vi "start.vi"(8 "error in (no error)":errorcluster, 11 "control references in":T1) -> (0 "error out":errorcluster, 3 "control references out":T1)   [LabVIEW 2010]
uses:
  type_definitions/clusters/controls_refs.ctl
  type_definitions/enumerations/main_control_types.ctl
  common/classes/GenericToplevelComponent/GenericToplevelComponent/GenericToplevelComponent.lvclass
  components/ImagingMode/GenericImagingMode/GenericImagingMode/GenericImagingMode.lvclass
  components/ExperimentController/GenericExperimentController/GenericExperimentController/GenericExperimentController.lvclass
  global_variables.vi
  common/classes/GenericComponent/GenericComponent/class_data.vi
  common/classes/GenericComponent/GenericComponent/GenericComponent.lvclass
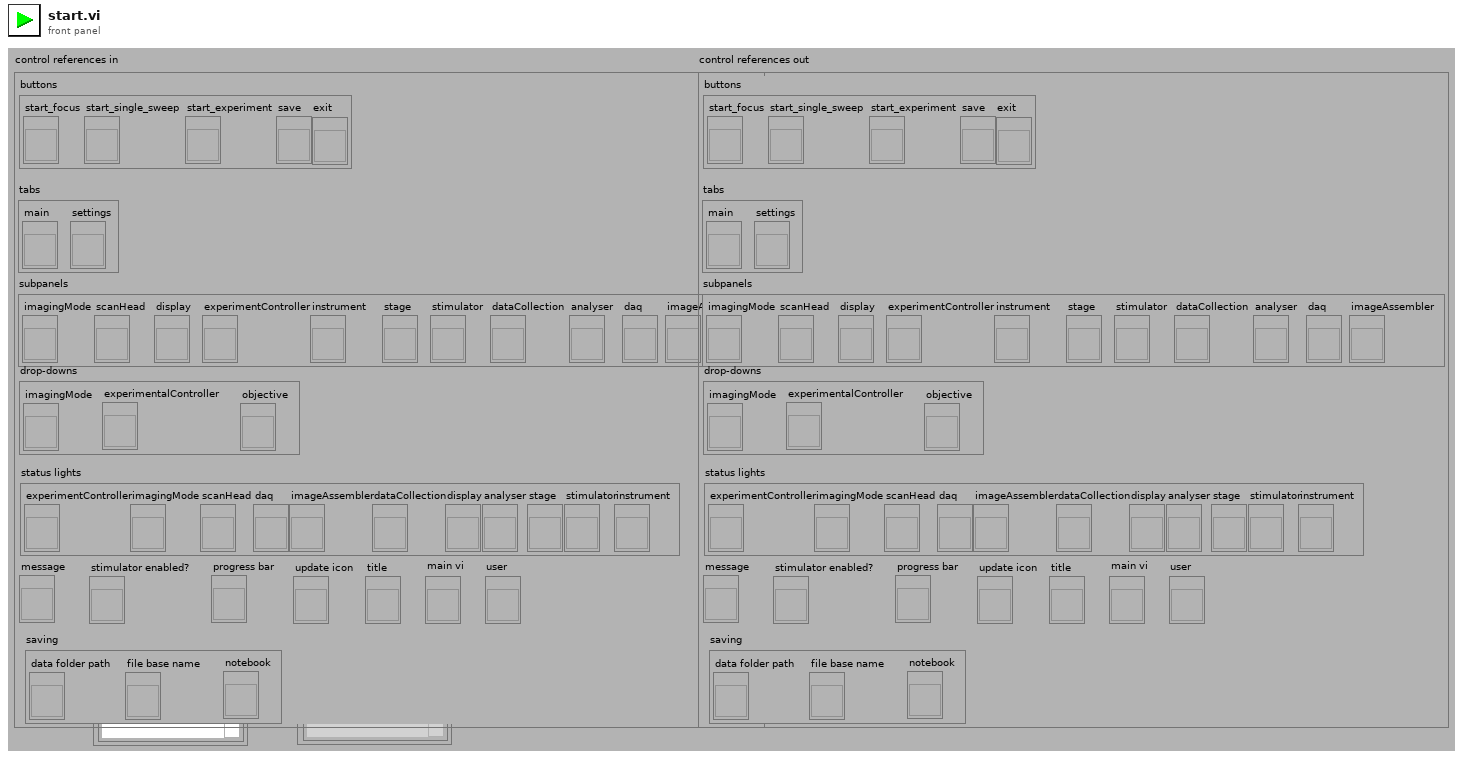
[diagram p1: front panel]
types:
  T1 = typedef "controls_refs.ctl" = cluster{"buttons":cluster{"start_focus":refnum<vi>, "start_single_sweep":refnum<vi>, "start_experiment":refnum<vi>, "save":refnum<vi>, "exit":refnum<vi>}, "tabs":cluster{"main":refnum<vi>, "settings":refnum<vi>}, "subpanels":cluster{"imagingMode":refnum<vi>, "scanHead":refnum<vi>, "display":refnum<vi>, "experimentController":refnum<vi>, "instrument":refnum<vi>, "stage":refnum<vi>, "stimulator":refnum<vi>, "dataCollection":refnum<vi>, "analyser":refnum<vi>, "daq":refnum<vi>, "imageAssembler":refnum<vi>}, "drop-downs":cluster{"imagingMode":refnum<vi>, "experimentalController":refnum<vi>, "objective":refnum<vi>}, "status lights":cluster{"experimentController":refnum<vi>, "imagingMode":refnum<vi>, "scanHead":refnum<vi>, "daq":refnum<vi>, "imageAssembler":refnum<vi>, "dataCollection":refnum<vi>, "display":refnum<vi>, "analyser":refnum<vi>, "stage":refnum<vi>, "stimulator":refnum<vi>, "instrument":refnum<vi>}, "message":refnum<vi>, "stimulator enabled?":refnum<vi>, "saving":cluster{"data folder path":refnum<vi>, "file base name":refnum<vi>, "notebook":refnum<vi>}, "progress bar":refnum<vi>, "update icon":refnum<vi>, "title":refnum<vi>, "main vi":refnum<vi>, "user":refnum<vi>}
  T2 = enum8{"Enabled", "Disabled", "Disabled and Grayed Out"}
  T3 = typedef "main_control_types.ctl" = enum16{"scan start button", "experimentController subpanel", "imagingMode subpanel", "scanHead subpanel", "dataCollection subpanel", "display subpanel", "analyser subpanel", "stimulator subpanel", "imagingMode drop-down", "experimentController drop-down", "objective drop-down", "exit button"}
  T4 = typedef "GenericToplevelComponent.lvclass/common_trigger_enum.ctl" = enum16{"NULL", "initialise", "terminate", "fetch command", "fetch data", "attach observer", "register as observer", "detach observer", "acknowledge", "start", "stop", "sweep started", "sweep finished", "experiment started", "experiment stopped"}
  T5 = typedef "run_mode_enum.ctl" = enum16{"focus mode", "single sweep mode", "experiment mode"}
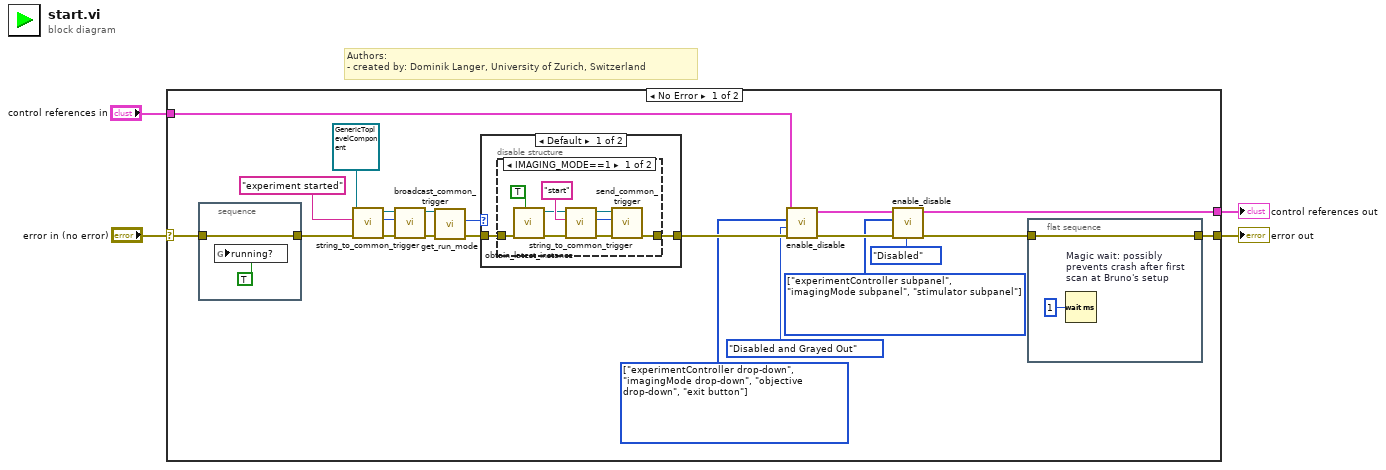
[diagram p0: block diagram]
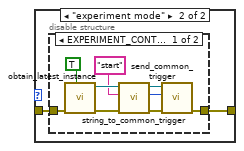
[diagram p3: hidden frame]
diagram:
  # "Authors: \n- created by: Dominik Langer, University of Zurich, Switzerland"
  n1 = case shown="No Error" "error in (no error)" {
    selector: "error in (no error)" -> [w24 w56]
    tunnel: [w20 w56] -> w3
    tunnel: "control references in" -> [w21 w55]
    tunnel: [w7 w55] -> w1
    frame No Error {
      w5 = T3[] [enum."experimentController subpanel", enum."imagingMode subpanel", enum."stimulator subpanel"] items=["scan start button", "experimentController subpanel", "imagingMode subpanel", "scanHead subpanel", "dataCollection subpanel", "display subpanel", "analyser subpanel", "stimulator subpanel", "imagingMode drop-down", "experimentController drop-down", "objective drop-down", "exit button"] ("controls")
      w11 = T3[] [enum."experimentController drop-down", enum."imagingMode drop-down", enum."objective drop-down", enum."exit button"] items=["scan start button", "experimentController subpanel", "imagingMode subpanel", "scanHead subpanel", "dataCollection subpanel", "display subpanel", "analyser subpanel", "stimulator subpanel", "imagingMode drop-down", "experimentController drop-down", "objective drop-down", "exit button"] ("controls")
      n2 = stacked-sequence {
        tunnel: w24 -> [w30]
        tunnel: [w30] -> w17
        frame #0 {
          n3 = global write "global_variables.vi" "running?"(TRUE) -> ()
        }
      }
      n4 = call-dynamic "string_to_common_trigger.vi"("error in (no error)"=w17, "trigger string"="experiment started", "GenericToplevelComponent in"=refnum<class "GenericToplevelComponent.lvclass"> refnum ("GenericToplevelComponent.lvclass")) -> ("error out"=w16:errorcluster, "trigger"=w15:T4, "GenericToplevelComponent out"=w14:refnum<class "GenericToplevelComponent.lvclass">)  [unwired: 6 in]
      n5 = call-dynamic "broadcast_common_trigger.vi"("error in (no error)"=w16, "trigger"=w15, "GenericToplevelComponent in"=w14) -> ("error out"=w19:errorcluster, "GenericToplevelComponent out"=w18:refnum<class "GenericToplevelComponent.lvclass">)  [unwired: 7 in]
      n6 = call "get_run_mode.vi"("error in (no error)"=w19, "GenericPlugin in"=w18) -> ("error out"=w26:errorcluster, "run mode"=w25:T5)  [unwired: 5 in, 3 out]
      n7 = case shown="Default" w25 {
        tunnel: [w32 w43] -> w23
        tunnel: w26 -> [w31 w44]
        frame Default {
          n8 = disable-structure shown="IMAGING_MODE==1" {
            disable-tunnel: w31 -> [w40 w42]
            disable-tunnel: [w41 w42] -> w32
            frame condition #0 (active) {
              n9 = call "obtain_latest_instance.vi"("quick, but maybe outdated?"=TRUE, "error in (no error)"=w40) -> ("error out"=w37:errorcluster, "GenericScanMode out"=w36:refnum<class "GenericImagingMode.lvclass">)  [unwired: 8 out]
              n10 = call-dynamic "string_to_common_trigger.vi"("error in (no error)"=w37, "trigger string"="start", "GenericToplevelComponent in"=w36) -> ("error out"=w33:errorcluster, "trigger"=w34:T4, "GenericToplevelComponent out"=w35:refnum<class "GenericImagingMode.lvclass">)  [unwired: 6 in]
              n11 = call-dynamic "send_common_trigger.vi"("error in (no error)"=w33, "trigger"=w34, "GenericToplevelComponent in"=w35) -> ("error out"=w41:errorcluster)  [unwired: 6 in, 2 out]
            }
            frame condition #1 {
            }
          }
        }
        frame "experiment mode" {
          n12 = disable-structure shown="EXPERIMENT_CONTROLLER==1" {
            disable-tunnel: w44 -> [w52 w54]
            disable-tunnel: [w51 w54] -> w43
            frame condition #0 (active) {
              n13 = call "obtain_latest_instance.vi"("quick, but maybe outdated?"=TRUE, "error in (no error)"=w52) -> ("error out"=w50:errorcluster, "GenericExperimentController out"=w49:refnum<class "GenericExperimentController.lvclass">)  [unwired: 8 in]
              n14 = call-dynamic "string_to_common_trigger.vi"("error in (no error)"=w50, "trigger string"="start", "GenericToplevelComponent in"=w49) -> ("error out"=w47:errorcluster, "trigger"=w46:T4, "GenericToplevelComponent out"=w48:refnum<class "GenericExperimentController.lvclass">)  [unwired: 6 in]
              n15 = call-dynamic "send_common_trigger.vi"("error in (no error)"=w47, "trigger"=w46, "GenericToplevelComponent in"=w48) -> ("error out"=w51:errorcluster)  [unwired: 6 in, 2 out]
            }
            frame condition #1 {
            }
          }
        }
      }
      n16 = call "enable_disable.vi"("error in (no error)"=w23, "state"=T2."Disabled and Grayed Out" ("Disabled"), "controls"=w11, "control references in"=w21) -> ("error out"=w10:errorcluster, "control references out"=w8:T1)  [unwired: 6 in]
      n17 = call "enable_disable.vi"("error in (no error)"=w10, "state"=T2."Disabled" ("Disabled"), "controls"=w5, "control references in"=w8) -> ("error out"=w9:errorcluster, "control references out"=w7:T1)  [unwired: 6 in]
      n18 = flat-sequence {
        tunnel: w9 -> [w27]
        tunnel: [w27] -> w20
        frame #0 {
          n19 = Wait (ms) "Magic wait: possibly prevents crash after first scan at Bruno's setup"(milliseconds to wait=u32 1) -> ()  [unwired: 1 out]
        }
      }
    }
    frame Error {
    }
  }
  "error out" <- w3
  "control references out" <- w1
